vi "Betriebsdaten Laden-Speichern.vi"(6 "Betriebsdaten":T2, 8 "Fehler (in)":errorcluster caption="Fehlerkonstante") -> (0 "error IO":errorcluster, 1 "Ausgangs-Cluster":T1)   [LabVIEW 2020, in "allgemeine Sub-VIs.lvlib"]
uses:
  allgemeine Sub-VIs.lvlib
  Betriebsdaten Aktionen.ctl
  Seiten/Gaszuordnung AO/FGV Gaszuordnung Gas-Auswahl Aktion.ctl
  Stoerungen/FGV Stoerung aufnehmen Aktion.ctl
  Stoerungen/FGV Stoermeldungen Aktion.ctl
  Seiten/Gaszuordnung AO/FGV Gaszuordnung Grenzen&Einheit Aktion.ctl
  Seiten/FT-IR/FGV FT-IR Aktionen.ctl
  AK-Schnittstelle/Aktionen Gespeicherte Werte.ctl
  Passwortverwaltung/FGV Passwort Aktion.ctl
  Seiten/Log Konfig/Aktionen Logdatei erstellen.ctl
  Seiten/Log Konfig/Aktionen Trigger.ctl
  cRIO/PC/Aktionen FGV Druckregler.ctl
  Seiten/FT-IR/Aktionen EVID-Codes.ctl
  Seiten/System Einstellungen V2/Aktioen FGV System.ctl
  Seiten/FT-IR/ReadLabFile/Aktionen Lab File.ctl
  Seiten/FT-IR/Algebraic Modul/FGV Algebraic Aktionen.ctl
  T90/Aktion FGV T90.ctl
  EPA 1065/ANR Test 1065-305/Aktion FGV ARN-Protokolleinstellungen.ctl
  EPA 1065/ANR Test 1065-305/Aktion FGV ARN Daten.ctl
  Seiten/FT-IR/Get Spectra/Aktion FGV Background-Daten.ctl
  Seiten/FT-IR/Aktion FGV Rezepte wechseln.ctl
  Seiten/CalGas Aufschaltung/FGV CalGas Aktionen.ctl
  Status Analysatoren/Aktion Status Analysatoren.ctl
  Auto Kalibrieren/KAL Daten loggen Aktionen.ctl
  Auto Kalibrieren/Aktionen FGV AutoKAL Daten.ctl
  Analysator Definition/FGV Analysator Definition Aktionen.ctl
  Linearisierung V2/Aktionen Polynom Daten speichern.ctl
  Linearisierung V2/Aktion Lin Daten aufarbeiten.ctl
  Linearisierung V2/Gasteiler/Aktionen FGV Gasteiler Daten.ctl
  Hangup Check/AktionFGV Hangup.ctl
  O2 Dichtheitstest/Aktion FGV O2 Leak.ctl
  Seiten/Grafik/Aktionen Konfig Diagramme.ctl
  PNS/Aktionen FGV Grenzwerte.ctl
  Auto Kalibrieren/Aktionen Zeitstempel speichern.ctl
  Seiten/System Einstellungen V2/Aktion FGV Gasbottledefinition.ctl
  Seiten/System Einstellungen V2/Aktion FGV SystemEinstellungenV2.ctl
  Seiten/System Einstellungen V2/Aktion FGV Gasdefinition.ctl
  Funktionstasten/Funktionstasten-Aktion.ctl
  Seiten/Anlagenuebersicht/VisBx Anzeige/Aktion FGV Ventile manuell schalten Crio.ctl
  Seiten/Log Konfig/Log Sequence FGV Aktion.ctl
  Seiten/FT-IR/FGV FT-IR Gasliste Aktionen.ctl
  Seiten/Erweiterte Konfig/Konfig CG-Check/Aktion_CG-Check.ctl
  Seiten/System Einstellungen V2/Aktioen FGV System Konstanten.ctl
  Seiten/EL3000/FID/FID Kalibrierung/Aktion FID Allgemeindaten.ctl
  Seiten/EL3000/FID/FID Kalibrierung/Aktionen FID Kal Komponente.ctl
  Amium PNS/Aktion FGV Amium Daten.ctl
  Seiten/Gaszuordnung AO/Gaszuordnung AO.lvlib
  Stoerungen/Stoerungen.lvlib
  Seiten/FT-IR/FT-IR.lvlib
  AK-Schnittstelle/AK-Schnittstelle.lvlib
  Passwortverwaltung/Passwort.lvlib
  Seiten/Log Konfig/LogKonfig.lvlib
  Seiten/Grafik/Grafik.lvlib
  cRIO/PC/Kommunikation mit cRIO.lvlib
  Seiten/System Einstellungen V2/System Einstellungen V2.lvlib
  Seiten/FT-IR/ReadLabFile/Read Lab File.lvlib
  Seiten/FT-IR/Algebraic Modul/Algebraic Modul.lvlib
  T90/T90.lvlib
  EPA 1065/ANR Test 1065-305/ARN Test 1065-305.lvlib
  Seiten/FT-IR/Get Spectra/Get Spectra.lvlib
  Seiten/EL3000/FID/FID.lvlib
  Seiten/EL3000/FID/FID Kalibrierung/FID Kalibrierung.lvlib
  Seiten/EL3000/FID/Aktion STY_MES.ctl
  Analysator Definition/Analysator Definition.lvlib
  Seiten/CalGas Aufschaltung/CalGas Aufschaltung.lvlib
  Status Analysatoren/Status Analysatoren.lvlib
  Auto Kalibrieren/Auto Kalibrieren.lvlib
  Seiten/Erweiterte Konfig/Konfig CG-Check/CG-Check Konfig.lvlib
  Amium PNS/Amium PNS.lvlib
  Linearisierung V2/Linearisierung v2.lvlib
  Linearisierung V2/Gasteiler/Gasteiler.lvlib
  Hangup Check/Hangup Check.lvlib
  O2 Dichtheitstest/O2 Dichtheitstest.lvlib
  PNS/PNS.lvlib
  Funktionstasten/Funktionstasten.lvlib
  Seiten/Anlagenuebersicht/VisBx Anzeige/Anlagenuebersicht.lvlib
  Seiten/CAN Konfig/CAN Konfig.lvlib
  Seiten/CAN Konfig/Aktion FGV CAN.ctl
  Seiten/CAN Konfig/Aktion FGV CAN2.ctl
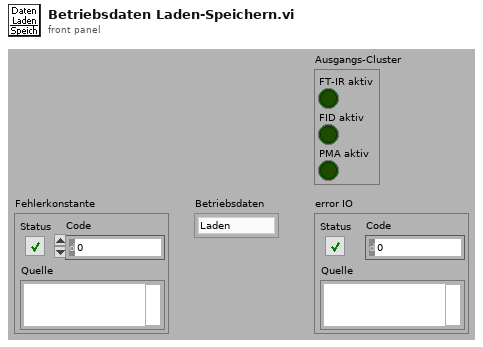
[diagram p1: front panel]
types:
  T1 = cluster{"FT-IR aktiv":bool, "FID aktiv":bool, "PMA aktiv":bool}
  T2 = typedef "allgemeine Sub-VIs.lvlib/Betriebsdaten Aktionen.ctl" = enum16{"Laden", "Speichern"}
  T3 = typedef "Anlagenuebersicht.lvlib/Aktion FGV Ventile manuell schalten Crio.ctl" = enum16{"lesen", "Ventile schalten", "Testbetrieb aktiv", "Testbetrieb inaktiv", "Anzeige Ventilstellung"}
  T4 = typedef "Funktionstasten.lvlib/Funktionstasten-Aktion.ctl" = enum16{"Initialisieren", "Zustand setzen", "Taste gedrückt", "Fehler speichern", "Lesen", "Manuell", "Remote", "Bitparallel", "Samplepoint", "Zeit Prüfen", "reset Umschalten"}
  T5 = typedef "System Einstellungen V2.lvlib/Aktion FGV Gasdefinition.ctl" = enum16{"lesen", "schreiben", "löschen", "laden", "speichern"}
  T6 = typedef "System Einstellungen V2.lvlib/Aktion FGV SystemEinstellungenV2.ctl" = enum16{"lesen", "Analysatoren schreiben", "Analysator ändern", "Analysatoren löschen", "laden", "speichern", "Untertitel", "Analysatoren", "Neue Analysatoren", "Gasteiler schreiben", "Gasteiler ändern", "Gasteiler löschen", "Gasteiler", "Gasteiler exportieren", "Gasteiler importieren"}
  T7 = typedef "System Einstellungen V2.lvlib/Aktion FGV Gasbottledefinition.ctl" = enum16{"lesen", "schreiben", "löschen", "laden", "speichern", "exportieren", "importieren"}
  T8 = typedef "Auto Kalibrieren.lvlib/Aktionen Zeitstempel speichern.ctl" = enum16{"lesen", "Zeitstempel NEU", "laden", "speichern"}
  T9 = typedef "PNS.lvlib/Aktionen FGV Grenzwerte.ctl" = enum16{"lesen", "Grenzw. schreiben", "Anweisungscode", "IP-Adresse", "laden", "speichern", "Anweisungscode vorgeben"}
  T10 = typedef "Grafik.lvlib/Aktionen Konfig Diagramme.ctl" = enum16{"lesen", "laden", "speichern", "X Auto Scale", "Y Auto Scale", "Anzeigedauer", "Y MIN", "Y MAX", "Referenzen", "Werteanzahl", "Autoscale einzeln"}
  T11 = typedef "LogKonfig.lvlib/Aktionen Logdatei erstellen.ctl" = enum16{"lesen", "Logdatei erstellen NEU", "Name NEU", "Pfad NEU", "Log Stop", "max Size"}
  T12 = typedef "O2 Dichtheitstest.lvlib/Aktion FGV O2 Leak.ctl" = enum16{"lesen", "O2 settings", "Pfad", "Protokoll", "laden", "speichern"}
  T13 = typedef "Hangup Check.lvlib/AktionFGV Hangup.ctl" = enum16{"lesen", "Hangup Settings", "Protokoll", "Pfad", "laden", "speichern"}
  T14 = typedef "Linearisierung v2.lvlib/Aktion Lin Daten aufarbeiten.ctl" = enum16{"lesen", "Protkolldaten", "speichern", "laden", "EPA auswerten", "Tabelle schreiben", "Lin auswerten", "Tab init", "Stufentabelle", "EPA aktiviert", "Nachbehandlung laden", "Tabelle löschen", "Istwerte löschen", "Zeile löschen", "Zeile einfügen", "LIN aktiviert", "LIN/EPA aktiv laden", "EGAK Tab", "LIN übernehmen", "Tab init ohne Stufen"}
  T15 = typedef "Linearisierung V2.lvlib/Gasteiler.lvlib/Aktionen FGV Gasteiler Daten.ctl" = enum16{"lesen", "Gasteiler Daten", "Seriellen Param.", "MB-Endwert", "laden", "speichern", "Anforderung", "TCP", "Aufzeichnung Start"}
  T16 = typedef "Linearisierung v2.lvlib/Aktionen Polynom Daten speichern.ctl" = enum16{"lesen", "laden", "speichern", "schreiben", "schreiben alle", "Liste erstellen", "aktivieren", "deaktivieren", "aktiv abfragen"}
  T17 = typedef "Analysator Definition.lvlib/FGV Analysator Definition Aktionen.ctl" = enum16{"lesen", "MB setzen", "MB KAL setzen", "laden"}
  T18 = typedef "Auto Kalibrieren.lvlib/Aktionen FGV AutoKAL Daten.ctl" = enum16{"lesen", "laden", "speichern", "Aufschaltzeit"}
  T19 = typedef "Auto Kalibrieren.lvlib/KAL Daten loggen Aktionen.ctl" = enum16{"lesen", "initialisieren", "loggen"}
  T20 = typedef "Status Analysatoren.lvlib/Aktion Status Analysatoren.ctl" = enum16{"lesen", "initialisieren", "Analysatoren aktiv", "FTIR Fehler", "FID Fehler", "PMA Fehler", "Felder einfärben"}
  T21 = typedef "CalGas Aufschaltung.lvlib/FGV CalGas Aktionen.ctl" = enum16{"lesen", "Analysator Auswahl", "Def.CalGas", "Aufschaltung CalGas", "laden", "speichern", "KAL extrahieren"}
  T22 = typedef "FT-IR.lvlib/Aktion FGV Rezepte wechseln.ctl" = enum16{"lesen", "Rezepte", "Rezeptindex", "Diesel", "Gasoline", "NCG", "laden", "speichern", "AK/Man"}
  T23 = typedef "FT-IR.lvlib/Get Spectra.lvlib/Aktion FGV Background-Daten.ctl" = enum16{"lesen", "schreiben", "Background aktiv", "Referenz", "laden", "speichern", "Plot sichtbar"}
  T24 = typedef "EPA 1065.lvlib/ARN Test 1065-305.lvlib/Aktion FGV ARN Daten.ctl" = enum16{"Lesen", "laden", "speichern", "ARN Daten", "Rohdaten", "Rohdaten löschen", "Zeitstempel", "SNR Ergebnis"}
  T25 = typedef "EPA 1065.lvlib/ARN Test 1065-305.lvlib/Aktion FGV ARN-Protokolleinstellungen.ctl" = enum16{"lesen", "schreiben", "laden", "speichern"}
  T26 = typedef "T90.lvlib/Aktion FGV T90.ctl" = enum16{"lesen", "schreiben", "laden", "speichern", "T90 aktiv", "T90 Entnahme aktiv", "Overflow Leak", "Pfad", "Zustand", "max. Responsetime"}
  T27 = typedef "FT-IR.lvlib/Algebraic Modul.lvlib/FGV Algebraic Aktionen.ctl" = enum16{"lesen", "laden", "speichern", "berechnen", "schreiben"}
  T28 = typedef "FT-IR.lvlib/Read Lab File.lvlib/Aktionen Lab File.ctl" = enum16{"lesen", "laden"}
  T29 = typedef "System Einstellungen V2.lvlib/Aktioen FGV System.ctl" = enum16{"lesen", "laden", "speichern", "Optionen schreiben", "Zeitstempel", "Reset BMP", "Reset SQP", "Wartung", "Werkseinstellung"}
  T30 = typedef "FT-IR.lvlib/Aktionen EVID-Codes.ctl" = enum16{"lesen", "setzen", "laden", "speichern", "1Hz/5Hz", "Smoothing", "Rolling Average"}
  T31 = typedef "Kommunikation mit cRIO.lvlib/Aktionen FGV Druckregler.ctl" = enum16{"lesen", "Parameter", "Istwerte", "laden", "speichern"}
  T32 = typedef "LogKonfig.lvlib/Aktionen Trigger.ctl" = enum16{"lesen", "ALLE schreiben", "Trigger prüfen", "Trigger rücksetzen"}
  T33 = typedef "Passwort.lvlib/FGV Passwort Aktion.ctl" = enum16{"prüfen", "setzen", "Initialisieren", "PW speichern", "lesen", "PW Änderung"}
  T34 = typedef "AK-Schnittstelle.lvlib/Aktionen Gespeicherte Werte.ctl" = enum16{"lesen", "laden", "speichern", "Seriell", "TCP", "Diverse", "AKTIV", "AK-Namen"}
  T35 = typedef "FT-IR.lvlib/FGV FT-IR Aktionen.ctl" = enum16{"lesen", "NOG setzen", "NOS setzen", "Initialisieren", "speichern", "ALLES setzen", "FT-IR Spektrum loggen", "Komm Stoppen", "Spektrum LogKonfig"}
  T36 = typedef "Gaszuordnung AO.lvlib/FGV Gaszuordnung Grenzen&Einheit Aktion.ctl" = enum16{"Lesen", "Schreiben Min", "Schreiben Max", "Laden", "Speichern"}
  T37 = typedef "Stoerungen.lvlib/FGV Stoermeldungen Aktion.ctl" = enum16{"Initialisieren", "kommend", "gehend", "lesen", "Queue leeren", "Queue freigeben", "in Datei loggen", "Änderung zurücksetzen"}
  T38 = typedef "Stoerungen.lvlib/FGV Stoerung aufnehmen Aktion.ctl" = enum16{"Initialisieren", "Schreiben", "Lesen", "Quittieren", "quit. löschen"}
  T39 = typedef "Gaszuordnung AO.lvlib/FGV Gaszuordnung Gas-Auswahl Aktion.ctl" = enum16{"Lesen", "AO Auswahl", "Graph Auswahl", "aktiver Graph", "laden", "speichern"}
  T40 = typedef "CAN Konfig.lvlib/Aktion FGV CAN.ctl" = enum16{"lesen", "schreiben Konfig", "Status", "Messdaten", "laden", "speichern", "CAN Data"}
  T41 = typedef "CAN Konfig.lvlib/Aktion FGV CAN2.ctl" = enum16{"lesen", "schreiben Konfig", "Status", "Messdaten", "laden", "speichern", "CAN Data", "reset more Frames avalable"}
  T42 = typedef "ABB-EL3000.lvlib/FID.lvlib/FID Kalibrierung.lvlib/Aktionen FID Kal Komponente.ctl" = enum16{"lesen", "setzen", "laden", "speichern", "LIN"}
  T43 = typedef "Aktion STY_MES.ctl" = enum16{"lesen", "setze STY", "setze MES", "MODBUS schreiben"}
  T44 = typedef "ABB-EL3000.lvlib/FID.lvlib/FID Kalibrierung.lvlib/Aktion FID Allgemeindaten.ctl" = enum16{"lesen", "Mod", "Time", "laden", "speichern"}
  T45 = typedef "Amium PNS.lvlib/Aktion FGV Amium Daten.ctl" = enum16{"lesen", "Komm Daten", "Daten", "Error", "Regler", "Grenzwerte", "laden", "speichern"}
  T46 = typedef "LogKonfig.lvlib/Log Sequence FGV Aktion.ctl" = enum16{"initialisieren", "lesen", "schreiben", "laden", "speichern", "übertragen"}
  T47 = typedef "FT-IR.lvlib/FGV FT-IR Gasliste Aktionen.ctl" = enum16{"lesen", "Gasliste FT-IR", "Gasliste ausgelesen", "laden", "speichern", "löschen"}
  T48 = typedef "Erweiterte Konfig.lvlib/CG-Check Konfig.lvlib/Aktion_CG-Check.ctl" = enum16{"lesen", "schreiben", "laden", "Komponente", "Aktive?", "speichern"}
  T49 = typedef "System Einstellungen V2.lvlib/Aktioen FGV System Konstanten.ctl" = enum16{"lesen", "laden", "speichern", "Sprache"}
  T50 = typedef "Analysator Definition.lvlib/Betriebsdaten Komponente.ctl" = cluster{"Namen":string[], "MB Namen":string[], "Einheit":string, "MB Aktuell":u16, "MB Endwert":u16, "CalGase":u16[], "MB für KAL":u16[], "CG für KAL":u16[]}
  T51 = typedef "Status Analysatoren.lvlib/Status.ctl" = cluster{"FT-IR aktiv":bool, "FT-IR Fehler":bool, "FID aktiv":bool, "FID Fehler":bool, "PMA aktiv":bool, "PMA Fehler":bool}
  T52 = typedef "LogKonfig.lvlib/Auswahlfeld aktiviert-deaktiviert.ctl" = u16
  T53 = typedef "LogKonfig.lvlib/Element Triggerereignisse.ctl" = cluster{"Trigger verwenden":T52, "Messwert":u16, "kl./gr.":u16, "Wert":sgl, "Puffergröße":sgl}
  T54 = cluster{"Status Analysatoren":T51, "max. Größe  in Byte neu":i64, "Logdatei erstellen neu":T52, "Name Log Datei neu":string, "Pfad LogDatei neu":path, "Triggerereignis neu":T53, u16[], "Samplepoint":u16}
  T55 = typedef "Linearisierung v2.lvlib/Polynome.ctl" = cluster{"Namen":string[], "Polynom":dbl[][], "Aktiv":bool[]}
  T56 = cluster{"FT-IR aktiv":bool, bool, "PMA aktiv":bool}
  T57 = cluster{"FT-IR aktiv":bool, "FID aktiv":bool, bool}
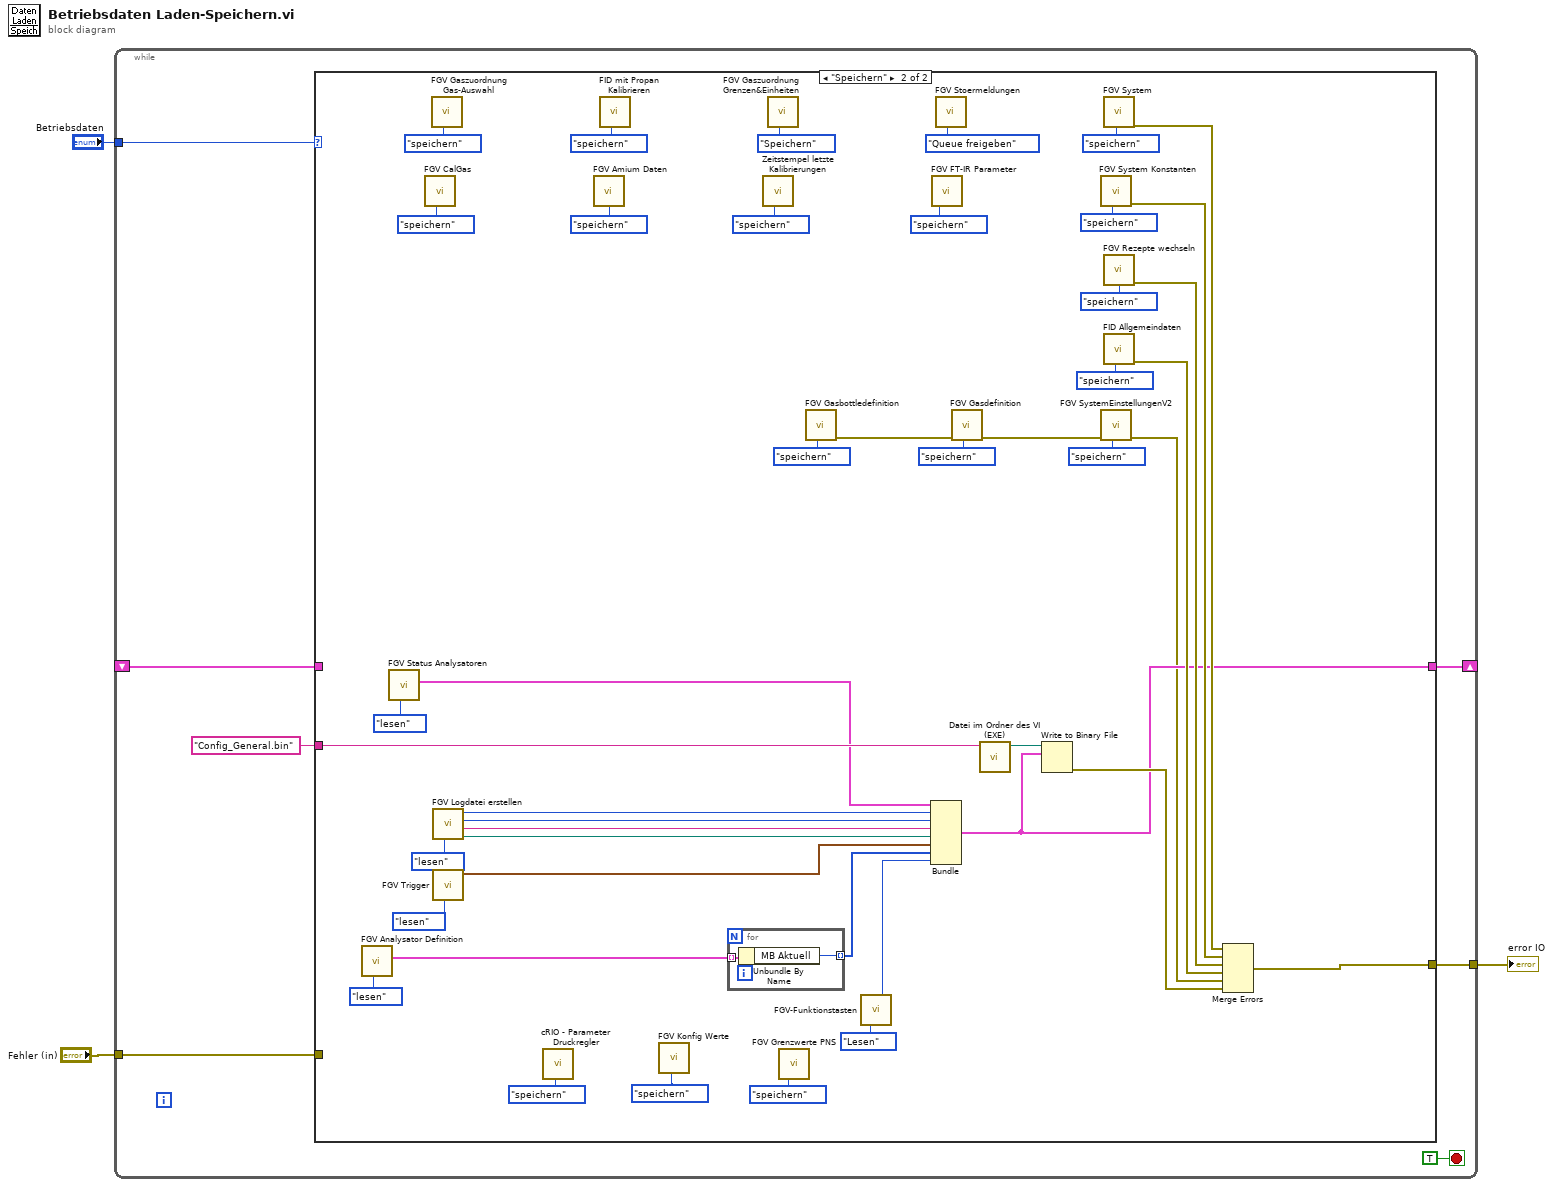
[diagram p0: block diagram]
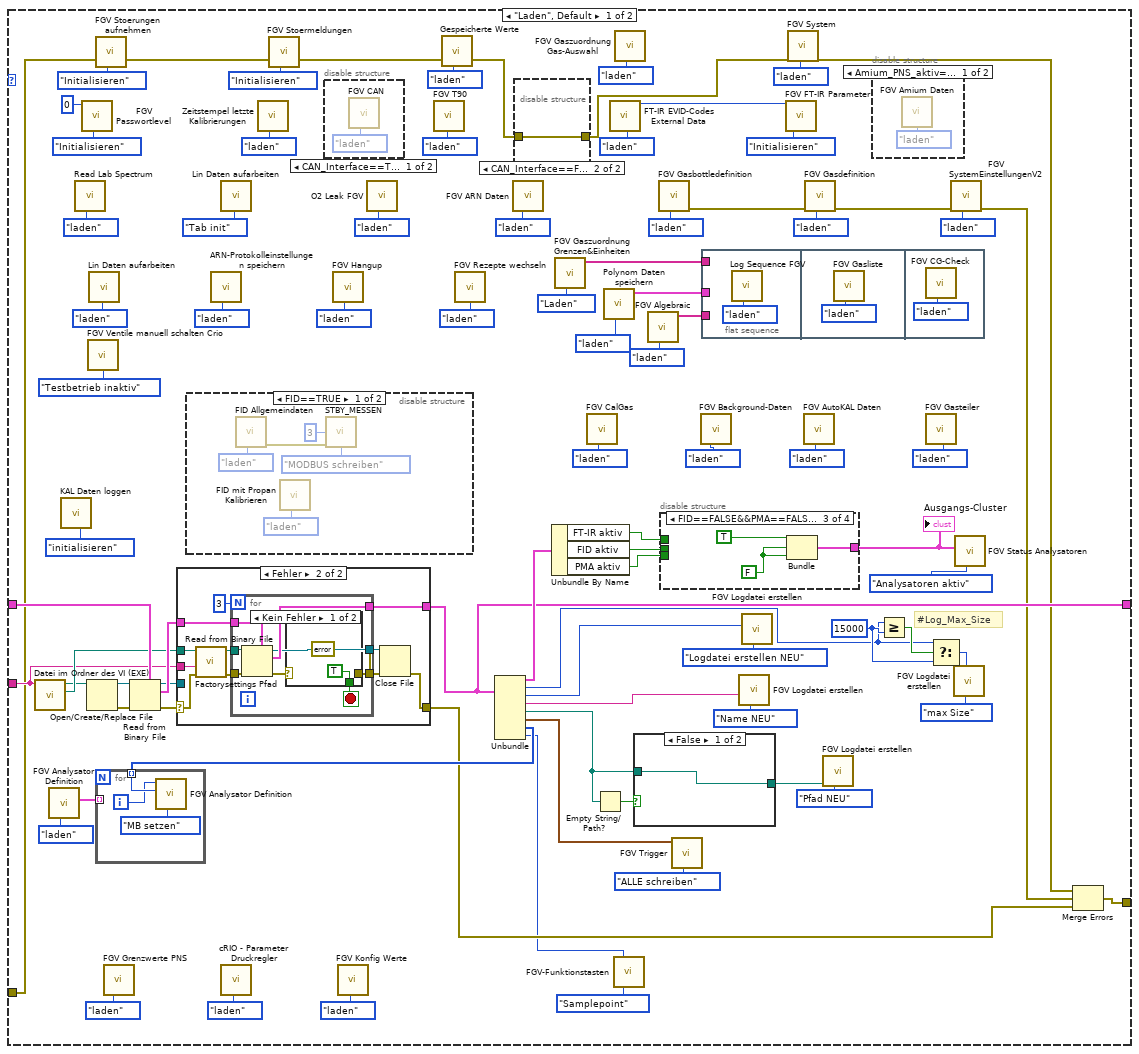
[diagram p2: hidden frame]
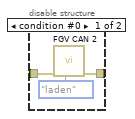
[diagram p4: hidden frame]
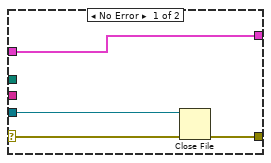
[diagram p7: hidden frame]
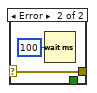
[diagram p8: hidden frame]
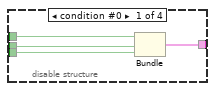
[diagram p9: hidden frame]
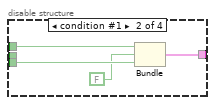
[diagram p10: hidden frame]
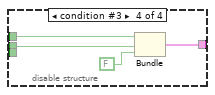
[diagram p11: hidden frame]
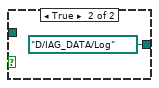
[diagram p12: hidden frame]
diagram:
  n1 = while {
    tunnel: "Betriebsdaten" -> [w9]
    shift-right: [w7] -> _
    shift-left: _ -> [w6]
    tunnel: "Fehler (in)" -> [w5]
    tunnel: [w4] -> w1
    stop <- TRUE stop-if-true
    n2 = case shown="\"Speichern\"" w9 {
      tunnel: "Config_General.bin" ("Dateiname") -> [w33 w197]
      tunnel: [w30 w165] -> w7
      tunnel: w6 -> [w85 _]
      tunnel: w5 -> [w12 _]
      tunnel: [w54 w174] -> w4
      frame "Laden", Default {
        w38 = i64 15000 ("y")
        # "#Log_Max_Size"
        n3 = call "Datei im Ordner des VI (EXE).vi"("Dateiname"=w33) -> ("Ordner des Haupt-VIs"=w34:path, "Dateipfad im Ordner des Haupt-VIs"=w25:path)  [unwired: 8 in, 1 out]
        n4 = call "FGV Analysator Definition.vi"("Aktionen"=FGV_Analysator_Definition_Aktionen."laden") -> ("Betriebsdaten"=w55:T50[])  [unwired: 6 in, 4 out]
        n5 = call "KAL Daten loggen.vi"("Aktionen MFC loggen"=KAL_Daten_loggen_Aktionen."initialisieren") -> ()  [unwired: 10 in, 1 out]
        n6 = call "Read Lab Spectrum.VI"("Aktionen"=Aktionen_Lab_File."laden") -> ()  [unwired: 7 in, 4 out]
        n7 = call "FGV Passwortlevel.vi"("FGV Passwort Aktion"=FGV_Passwort_Aktion."Initialisieren", "geforderter Level"=i16 0) -> ()  [unwired: 2 in, 8 out]
        n8 = Open/Create/Replace File(file path (use dialog)=w25) -> (refnum out=w24:refnum<file>, error out=w26:errorcluster)  [unwired: 5 in, 1 out]
        n9 = call "FGV Ventile manuell schalten Crio.vi"("Aktion"=Aktion_FGV_Ventile_manuell_schalten_Crio."Testbetrieb inaktiv") -> ()  [unwired: 11 in, 4 out]
        n10 = call "Lin Daten aufarbeiten.vi"("Aktionen"=Aktion_Lin_Daten_aufarbeiten."laden") -> ()  [unwired: 16 in, 11 out]
        n11 = call "FGV Stoerungen aufnehmen.vi"("FGV Störung aufnehmen Aktion"=FGV_Stoerung_aufnehmen_Aktion."Initialisieren" ("FGV Störung Aktion")) -> ()  [unwired: 2 in, 9 out]
        n12 = call "FGV Grenzwerte PNS.vi"("Aktionen FGV Grenzwerte"=Aktionen_FGV_Grenzwerte."laden") -> ()  [unwired: 12 in, 3 out]
        n13 = Read from Binary File(5:w85, 8:w26, 11:w24) -> (0:w31:errorcluster, 2:w35:T54, 3:w32:refnum<file>)  [unwired: 4 out]
        n14 = case shown="Fehler" w31 {
          selector: w31 -> [w106 w110]
          tunnel: w34 -> [_ w111]
          tunnel: w35 -> [w107 w109]
          tunnel: [w107 w117] -> w30
          tunnel: [w104 w115] -> w29
          tunnel: w32 -> [w105 _]
          tunnel: w33 -> [_ w108]
          frame No Error {
            n15 = Close File(refnum=w105, error in=w106) -> (error out=w104:errorcluster)  [unwired: 1 out]
          }
          frame Error {
            n16 = call "Factorysettings Pfad.vi"("error in (no error)"=w110, "Dateiname"=w108, "Ordner des Haupt-VIs"=w111) -> ("error out"=w112:errorcluster, "Pfad Factorysettings"=w113:path)  [unwired: 7 in]
            n17 = for {
              N: 3 -> [_]
              tunnel: w112 -> [w124]
              tunnel: w113 -> [w123]
              tunnel: [w122] -> w117
              tunnel: [w121] -> w116
              tunnel: [w120] -> w114
              tunnel: w109 -> [w119]
              stop <- w125 stop-if-true
              n18 = Read from Binary File(5:w119, 8:w124, 11:w123) -> (0:w126:errorcluster, 2:w122:T54, 3:w120:refnum<file>)  [unwired: 3 in, 1 out]
              n19 = case shown="Kein Fehler" w126 {
                selector: w126 -> [_ w129]
                tunnel: [TRUE _] -> w125
                tunnel: [errorcluster {"status"=FALSE, "code"=0, "source"=""} ("error IO") w129] -> w121
                frame No Error {
                }
                frame Error {
                  n20 = Wait (ms)(milliseconds to wait=u32 100 ("Zu wartende ms")) -> ()  [unwired: 1 out]
                }
              }
            }
            n21 = Close File(refnum=w114, error in=w116) -> (error out=w115:errorcluster)  [unwired: 1 out]
          }
        }
        n22 = disable-structure shown="FID==TRUE" {
          frame condition #0 {
            n23 = call "FID Allgemeindaten.vi"("Aktion"=Aktion_FID_Allgemeindaten."laden") -> ("error out"=w101:errorcluster)  [unwired: 9 in, 1 out]
            n24 = call "FID mit Propan Kalibrieren.vi"("Aktionen"=Aktionen_FID_Kal_Komponente."laden") -> ()  [unwired: 9 in, 2 out]
            n25 = call "STBY_MESSEN.vi"("Case Nr."=3, "error in (no error)"=w101, "Aktion"=Aktion_STY_MES."MODBUS schreiben") -> ()  [unwired: 9 in, 4 out]
          }
          frame condition #1 (active) {
          }
        }
        n26 = call "ARN-Protokolleinstellungen speichern.vi"("Aktion"=Aktion_FGV_ARN-Protokolleinstellungen."laden") -> ()  [unwired: 9 in, 2 out]
        n27 = call "Lin Daten aufarbeiten.vi"("Aktionen"=Aktion_Lin_Daten_aufarbeiten."Tab init") -> ()  [unwired: 16 in, 11 out]
        n28 = call "cRIO - Parameter Druckregler.vi"("Aktion"=Aktionen_FGV_Druckregler."laden") -> ()  [unwired: 9 in, 10 out]
        n29 = call "Zeitstempel letzte Kalibrierungen.vi"("Aktionen"=Aktionen_Zeitstempel_speichern."laden") -> ()  [unwired: 10 in, 1 out]
        n30 = call "FGV Stoermeldungen.vi"("Aktion"=FGV_Stoermeldungen_Aktion."Initialisieren") -> ()  [unwired: 3 in, 8 out]
        n31 = disable-structure shown="CAN_Interface==TRUE, Standard" {
          frame condition #0 {
            n32 = call "FGV CAN.vi"("Aktion"=Aktion_FGV_CAN."laden") -> ()  [unwired: 6 in, 5 out]
          }
          frame condition #1 (active) {
          }
        }
        n33 = call "FGV Hangup.vi"("Aktion"=AktionFGV_Hangup."laden") -> ()  [unwired: 6 in, 5 out]
        n34 = call "FGV Konfig Werte.vi"("Aktionen"=Aktionen_Konfig_Diagramme."laden" ("Aktionen Konfig Diagramme")) -> ()  [unwired: 10 in, 9 out]
        n35 = call "O2 Leak FGV.vi"("Aktion"=Aktion_FGV_O2_Leak."laden") -> ()  [unwired: 6 in, 5 out]
        n36 = call "FGV T90.vi"("Aktion"=Aktion_FGV_T90."laden") -> ()  [unwired: 20 in, 7 out]
        n37 = call "Gespeicherte Werte.vi"("Aktionen"=Aktionen_Gespeicherte_Werte."laden") -> ()  [unwired: 6 in, 5 out]
        n38 = call "FGV Rezepte wechseln.vi"("Aktion"=Aktion_FGV_Rezepte_wechseln."laden") -> ()  [unwired: 8 in, 7 out]
        n39 = Unbundle(w30) -> ("Status Analysatoren"=w46:T51, "max. Größe  in Byte neu"=w37:i64, "Logdatei erstellen neu"=w41:T52, "Name Log Datei neu"=w42:string, "Pfad LogDatei neu"=w43:path, "Triggerereignis neu"=w44:T53, w45:u16[], "Samplepoint"=w14:u16)
        n40 = for {
          tunnel: w45 -> [w132] mode=indexing
          tunnel: w55 -> [_] mode=indexing
          i -> [w131]
          n41 = call "FGV Analysator Definition.vi"("Aktionen"=FGV_Analysator_Definition_Aktionen."MB setzen", "Messbereich"=w132, "Komponente"=w131) -> ()  [unwired: 4 in, 5 out]
        }
        n42 = call "FGV ARN Daten.vi"("Aktion"=Aktion_FGV_ARN_Daten."laden") -> ()  [unwired: 9 in, 6 out]
        n43 = disable-structure shown="CAN_Interface==FALSE" {
          disable-tunnel: w12 -> [w95 w97]
          disable-tunnel: [w94 w97] -> w11
          frame condition #0 {
            n44 = call "FGV CAN 2.vi"("Aktion"=Aktion_FGV_CAN2."laden", "error in (no error)"=w95) -> ("error out"=w94:errorcluster)  [unwired: 4 in, 5 out]
          }
          frame condition #1 (active) {
          }
        }
        n45 = Unbundle By Name(w46) -> ("FT-IR aktiv"=w62:bool, "FID aktiv"=w61:bool, "PMA aktiv"=w60:bool)
        n46 = call "FGV Gaszuordnung Grenzen&Einheiten.vi"("Aktion"=FGV_Gaszuordnung_Grenzen&Einheit_Aktion."Laden") -> ("Namen neu"=w70:string[])  [unwired: 2 in, 8 out]
        n47 = call "FGV CalGas.vi"("Aktionen"=FGV_CalGas_Aktionen."laden") -> ()  [unwired: 6 in, 5 out]
        n48 = Empty String/Path?(string/path=w43) -> (empty?=w80:bool)
        n49 = call "Polynom Daten speichern.vi"("Aktionen"=Aktionen_Polynom_Daten_speichern."laden") -> ("Polynome"=w52:T55)  [unwired: 5 in, 5 out]
        n50 = call "FT-IR EVID-Codes External Data.vi"("Aktionen"=Aktionen_EVID-Codes."laden") -> ("Startadresse"=w69:i32)  [unwired: 9 in, 5 out]
        n51 = call "FGV-Funktionstasten.vi"("Samplepoint"=w14, "Aktion"=Funktionstasten-Aktion."Samplepoint") -> ()  [unwired: 6 in, 8 out]
        n52 = call "FGV Gaszuordnung Gas-Auswahl.vi"("Aktion"=FGV_Gaszuordnung_Gas-Auswahl_Aktion."laden") -> ()  [unwired: 3 in, 8 out]
        n53 = case shown="False" w80 {
          tunnel: w43 -> [w152 _]
          tunnel: [w152 path "D:/IAG_DATA/Log" ("Pfad LogDatei neu")] -> w79
          frame False {
          }
          frame True {
          }
        }
        n54 = call "FGV Algebraic.vi"("Aktionen Algebraic"=FGV_Algebraic_Aktionen."laden") -> ("Namen"=w71:string[])  [unwired: 6 in, 4 out]
        n55 = call "FGV Gasbottledefinition.vi"("Aktion"=Aktion_FGV_Gasbottledefinition."laden") -> ("error out"=w19:errorcluster)  [unwired: 8 in, 2 out]
        n56 = disable-structure shown="FID==FALSE&&PMA==FALSE, Standard" {
          disable-tunnel: w62 -> [w140 w144 _ w151]
          disable-tunnel: w61 -> [w139 _ _ w150]
          disable-tunnel: w60 -> [w138 w143 _ _]
          disable-tunnel: [w137 w142 w147 w149] -> w59
          frame condition #0 {
            n57 = Bundle("FT-IR aktiv"=w140, "FID aktiv"=w139, "PMA aktiv"=w138) -> (w137:T1)  [unwired: 1 in]
          }
          frame condition #1 {
            n58 = Bundle("FT-IR aktiv"=w144, FALSE, "PMA aktiv"=w143) -> (w142:T56)  [unwired: 1 in]
          }
          frame condition #2 (active) {
            w146 = FALSE
            n59 = Bundle(TRUE, w146, w146) -> (w147:cluster{bool, bool, bool})  [unwired: 1 in]
          }
          frame condition #3 {
            n60 = Bundle("FT-IR aktiv"=w151, "FID aktiv"=w150, FALSE) -> (w149:T57)  [unwired: 1 in]
          }
        }
        "Ausgangs-Cluster" <- w59
        n61 = call "FGV Trigger.vi"("Aktion"=Aktionen_Trigger."ALLE schreiben", "Triggerereignis"=w44) -> ()  [unwired: 6 in, 4 out]
        n62 = call "FGV Background-Daten.vi"("Aktion"=Aktion_FGV_Background-Daten."laden") -> ()  [unwired: 7 in, 8 out]
        n63 = flat-sequence {
          tunnel: w52 -> [_]
          tunnel: w70 -> [_]
          tunnel: w71 -> [_]
          frame #0 {
            n64 = call "Log Sequence FGV.vi"("Aktion"=Log_Sequence_FGV_Aktion."laden") -> ()  [unwired: 10 in, 1 out]
          }
          frame #1 {
            n65 = call "FGV Gasliste.vi"("Aktionen"=FGV_FT-IR_Gasliste_Aktionen."laden") -> ()  [unwired: 8 in, 3 out]
          }
          frame #2 {
            n66 = call "FGV CG-Check.vi"("Aktion"=Aktion_CG-Check."laden") -> ()  [unwired: 11 in, 8 out]
          }
        }
        n67 = call "FGV Logdatei erstellen.vi"("Aktion"=Aktionen_Logdatei_erstellen."Name NEU", "Name LogDatei"=w42) -> ()  [unwired: 5 in, 5 out]
        n68 = call "FGV Logdatei erstellen.vi"("Aktion"=Aktionen_Logdatei_erstellen."Logdatei erstellen NEU", "Logdatei erstellen"=w41) -> ()  [unwired: 5 in, 5 out]
        n69 = call "FGV FT-IR Parameter.vi"("NoOfGasses neu"=w69, "Aktion"=FGV_FT-IR_Aktionen."Initialisieren") -> ()  [unwired: 10 in, 8 out]
        n70 = call "FGV System.vi"("error in (no error)"=w11, "Aktionen"=Aktioen_FGV_System."laden") -> ("error out"=w17:errorcluster)  [unwired: 11 in, 6 out]
        n71 = call "FGV AutoKAL Daten.vi"("Aktionen"=Aktionen_FGV_AutoKAL_Daten."laden") -> ()  [unwired: 10 in, 1 out]
        n72 = call "FGV Gasdefinition.vi"("Aktion"=Aktion_FGV_Gasdefinition."laden", "error in (no error)"=w19) -> ("error out"=w18:errorcluster)  [unwired: 8 in, 1 out]
        n73 = call "FGV Logdatei erstellen.vi"("Aktion"=Aktionen_Logdatei_erstellen."Pfad NEU", "Pfad Log Datei"=w79) -> ()  [unwired: 5 in, 5 out]
        n74 = disable-structure shown="Amium_PNS_aktiv==TRUE, Standard" {
          frame condition #0 {
            n75 = call "FGV Amium Daten.vi"("Aktion"=Aktion_FGV_Amium_Daten."laden") -> ()  [unwired: 9 in, 6 out]
          }
          frame condition #1 (active) {
          }
        }
        n76 = Greater Or Equal?(x=w37, y=w38) -> (x >= y?=w39:bool)
        n77 = call "FGV Gasteiler.vi"("Aktionen"=Aktionen_FGV_Gasteiler_Daten."laden") -> ()  [unwired: 11 in, 8 out]
        n78 = Select(t=w37, s=w39, f=w38) -> (s? t:f=w36:i64)
        n79 = call "FGV SystemEinstellungenV2.vi"("Aktion"=Aktion_FGV_SystemEinstellungenV2."laden", "error in (no error)"=w18) -> ("error out"=w16:errorcluster)  [unwired: 4 in, 5 out]
        n80 = call "FGV Logdatei erstellen.vi"("Aktion"=Aktionen_Logdatei_erstellen."max Size", "max. Größe  in Byte"=w36) -> ()  [unwired: 5 in, 5 out]
        n81 = call "FGV Status Analysatoren.vi"("Aktionen"=Aktion_Status_Analysatoren."Analysatoren aktiv", "Aktiv"=w59) -> ()  [unwired: 9 in, 1 out]
        n82 = Merge Errors(w17, w16, w29) -> (w54:errorcluster)
      }
      frame "Speichern" {
        n83 = call "FGV Analysator Definition.vi"("Aktionen"=FGV_Analysator_Definition_Aktionen."lesen") -> ("Betriebsdaten"=w176:T50[])  [unwired: 6 in, 4 out]
        n84 = call "FGV Status Analysatoren.vi"("Aktionen"=Aktion_Status_Analysatoren."lesen") -> ("Status Analysatoren"=w167:T51)  [unwired: 10 in]
        n85 = call "FGV CalGas.vi"("Aktionen"=FGV_CalGas_Aktionen."speichern") -> ()  [unwired: 6 in, 5 out]
        n86 = call "FGV Gaszuordnung Gas-Auswahl.vi"("Aktion"=FGV_Gaszuordnung_Gas-Auswahl_Aktion."speichern") -> ()  [unwired: 3 in, 8 out]
        n87 = call "FGV Logdatei erstellen.vi"("Aktion"=Aktionen_Logdatei_erstellen."lesen") -> ("Pfad LogDatei neu"=w190:path, "Name Log Datei neu"=w191:string, "Logdatei erstellen neu"=w192:T52, "max. Größe  in Byte neu"=w166:i64)  [unwired: 6 in, 1 out]
        n88 = call "FGV Trigger.vi"("Aktion"=Aktionen_Trigger."lesen") -> ("Triggerereignis neu"=w189:T53)  [unwired: 7 in, 3 out]
        n89 = call "cRIO - Parameter Druckregler.vi"("Aktion"=Aktionen_FGV_Druckregler."speichern") -> ()  [unwired: 9 in, 10 out]
        n90 = call "FGV Amium Daten.vi"("Aktion"=Aktion_FGV_Amium_Daten."speichern") -> ()  [unwired: 9 in, 6 out]
        n91 = call "FID mit Propan Kalibrieren.vi"("Aktionen"=Aktionen_FID_Kal_Komponente."speichern") -> ()  [unwired: 9 in, 2 out]
        n92 = call "FGV Konfig Werte.vi"("Aktionen"=Aktionen_Konfig_Diagramme."speichern" ("Aktionen Konfig Diagramme")) -> ()  [unwired: 10 in, 9 out]
        n93 = for {
          tunnel: w176 -> [w199] mode=indexing
          tunnel: [w198] -> w175 mode=indexing
          n94 = Unbundle By Name(w199) -> ("MB Aktuell"=w198:u16)
        }
        n95 = call "Zeitstempel letzte Kalibrierungen.vi"("Aktionen"=Aktionen_Zeitstempel_speichern."speichern") -> ()  [unwired: 10 in, 1 out]
        n96 = call "FGV Gaszuordnung Grenzen&Einheiten.vi"("Aktion"=FGV_Gaszuordnung_Grenzen&Einheit_Aktion."Speichern") -> ()  [unwired: 2 in, 9 out]
        n97 = call "FGV Grenzwerte PNS.vi"("Aktionen FGV Grenzwerte"=Aktionen_FGV_Grenzwerte."speichern") -> ()  [unwired: 12 in, 3 out]
        n98 = call "FGV Gasbottledefinition.vi"("Aktion"=Aktion_FGV_Gasbottledefinition."speichern") -> ("error out"=w158:errorcluster)  [unwired: 8 in, 2 out]
        n99 = call "FGV-Funktionstasten.vi"("Aktion"=Funktionstasten-Aktion."Lesen") -> ("Samplepoint"=w154:u16)  [unwired: 7 in, 7 out]
        n100 = Bundle("Status Analysatoren"=w167, "max. Größe  in Byte neu"=w166, "Logdatei erstellen neu"=w192, "Name Log Datei neu"=w191, "Pfad LogDatei neu"=w190, "Triggerereignis neu"=w189, w175, "Samplepoint"=w154) -> (w165:T54)  [unwired: 1 in]
        n101 = call "FGV FT-IR Parameter.vi"("Aktion"=FGV_FT-IR_Aktionen."speichern") -> ()  [unwired: 11 in, 8 out]
        n102 = call "FGV Stoermeldungen.vi"("Aktion"=FGV_Stoermeldungen_Aktion."Queue freigeben") -> ()  [unwired: 3 in, 8 out]
        n103 = call "FGV Gasdefinition.vi"("Aktion"=Aktion_FGV_Gasdefinition."speichern", "error in (no error)"=w158) -> ("error out"=w157:errorcluster)  [unwired: 8 in, 1 out]
        n104 = call "Datei im Ordner des VI (EXE).vi"("Dateiname"=w197) -> ("Dateipfad im Ordner des Haupt-VIs"=w195:path)  [unwired: 8 in, 2 out]
        n105 = Write to Binary File(file (use dialog)=w195, data=w165) -> (error out=w169:errorcluster)  [unwired: 1 in, 5 out]
        n106 = call "FGV System Konstanten.vi"("Aktionen"=Aktioen_FGV_System_Konstanten."speichern") -> ("error out"=w172:errorcluster)  [unwired: 6 in, 4 out]
        n107 = call "FGV SystemEinstellungenV2.vi"("Aktion"=Aktion_FGV_SystemEinstellungenV2."speichern", "error in (no error)"=w157) -> ("error out"=w156:errorcluster)  [unwired: 4 in, 5 out]
        n108 = call "FGV System.vi"("Aktionen"=Aktioen_FGV_System."speichern") -> ("error out"=w173:errorcluster)  [unwired: 12 in, 6 out]
        n109 = call "FGV Rezepte wechseln.vi"("Aktion"=Aktion_FGV_Rezepte_wechseln."speichern") -> ("error out"=w171:errorcluster)  [unwired: 8 in, 6 out]
        n110 = call "FID Allgemeindaten.vi"("Aktion"=Aktion_FID_Allgemeindaten."speichern") -> ("error out"=w170:errorcluster)  [unwired: 9 in, 1 out]
        n111 = Merge Errors(w173, w172, w171, w170, w156, w169) -> (w174:errorcluster)
      }
    }
  }
  "error IO" <- w1
